vi "ROI Segment Points to Array of Pixels.vi"(8 "error in (no error)":errorcluster, 11 "Segment ROI Points":i32[](array[numeric])) -> (0 "Error Out":errorcluster, 1 "Number of Points":i32, 3 "Pixels of the Segment":cluster{"X":i32, "Y":i32}[](array[cluster]))   [LabVIEW 2021, in "Image.lvlib"]
uses:
  Image.lvlib
  <vilib>/vision/NI_Vision_Development_Module.lvlib
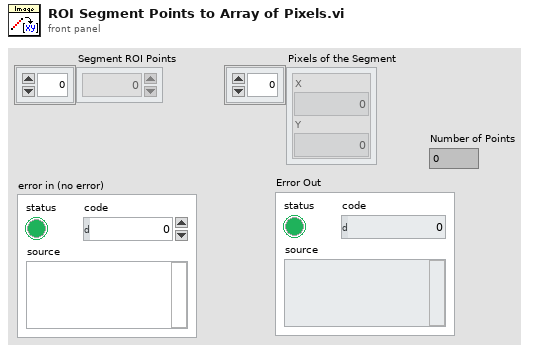
[diagram p1: front panel]
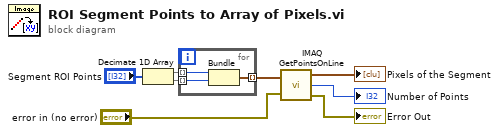
[diagram p0: block diagram]
diagram:
  n1 = Decimate 1D Array("Segment ROI Points") -> (w4:i32[], w5:i32[])
  n2 = for {
    tunnel: w4 -> [w11] mode=indexing
    tunnel: w5 -> [w10] mode=indexing
    tunnel: [w9] -> w6 mode=indexing
    n3 = Bundle("Numeric"=w11, "Numeric"=w10) -> (w9:cluster{"Numeric":i32, "Numeric":i32})  [unwired: 1 in]
  }
  n4 = call "IMAQ GetPointsOnLine"("Endpoints"=w6, "error in (no error)"="error in (no error)") -> ("Points of the Line"=→"Pixels of the Segment":cluster{"X":i32, "Y":i32}[], "Number of Points"=→"Number of Points":i32, "error out"=→"Error Out":errorcluster)
